vi "Log Binning.vi"(4 "Max Freq":dbl[unit]=1000000000.0 format="%#_6p", 5 "Number Elements":u32=200, 6 "Frequencies":dbl[](array[numeric]), 7 "Spectrum":dbl[](array[numeric])) -> (2 "Frequencies Binned":dbl[](array[numeric]), 3 "Spectrum Binned":dbl[](array[numeric]))   [LabVIEW 2010]
panel:
  out "Log Range":dbl[](array[numeric])=[nan, nan, nan, nan, nan, nan, nan, nan, nan, nan, nan, nan, nan, nan, nan, nan, nan, nan, nan, nan, nan, nan, nan, nan, nan, nan, nan, nan, nan, nan, nan, nan, nan, nan, nan, nan, nan, nan, nan, nan, nan, nan, nan, nan, nan, nan, nan, nan, nan, nan, nan, nan, nan, nan, nan, nan, nan, nan, nan, nan, nan, nan, nan, nan, nan, nan, nan, nan, nan, nan, nan, nan, nan, nan, nan, nan, nan, nan, nan, nan, nan, nan, nan, nan, nan, nan, nan, nan, nan, nan, nan, nan, nan, nan, nan, nan, nan, nan, nan, nan, nan, nan, nan, nan, nan, nan, nan, nan, nan, nan, nan, nan, nan, nan, nan, nan, nan, nan, nan, nan, nan, nan, nan, nan, nan, nan, nan, nan, nan, nan, nan, nan, nan, nan, nan, nan, nan, nan, nan, nan, nan, nan, nan, nan, nan, nan, nan, nan, nan, nan, nan, nan, nan, nan, nan, nan, nan, nan, nan, nan, nan, nan, nan, nan, nan, nan, nan, nan, nan, nan, nan, nan, nan, nan, nan, nan, nan, nan, nan, nan, nan, nan, nan, nan, nan, nan, nan, nan, nan, nan, nan, nan, nan, nan, nan, nan, nan, nan, nan, nan]
  out "XY Graph":cluster{dbl[], dbl[]}[](graph)
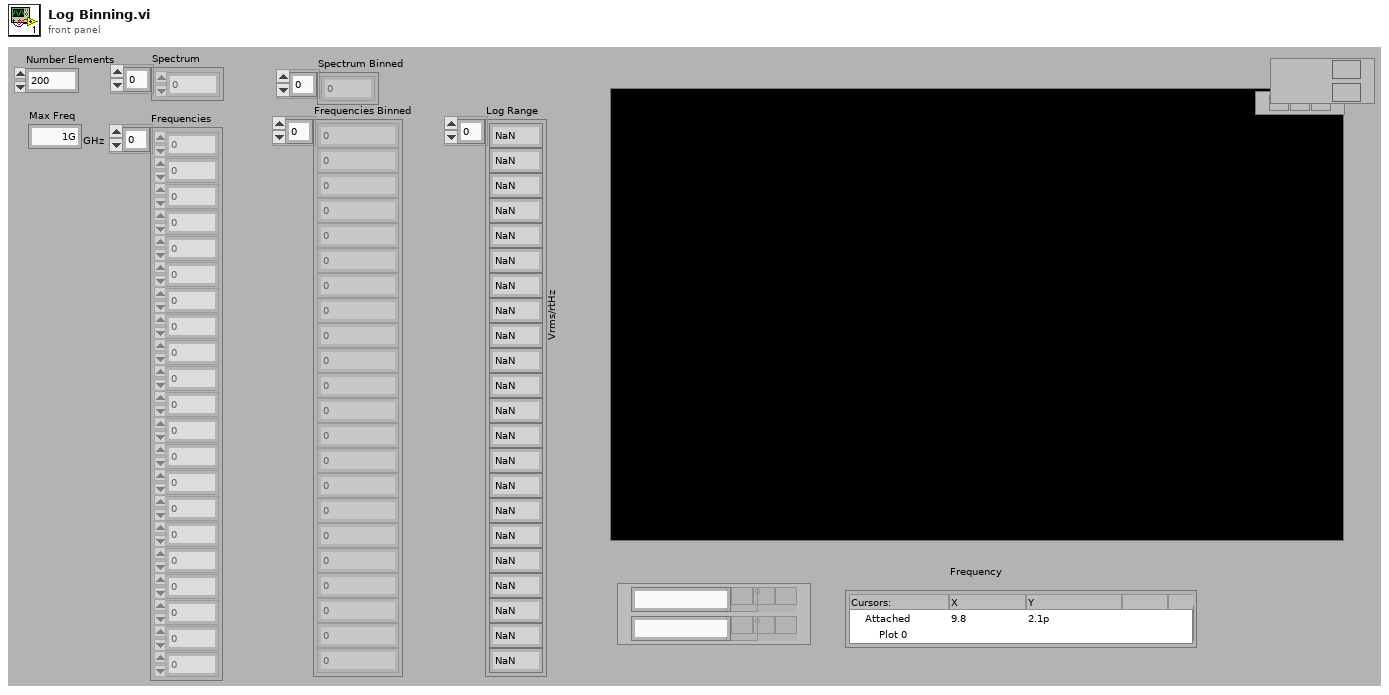
[diagram p1: front panel]
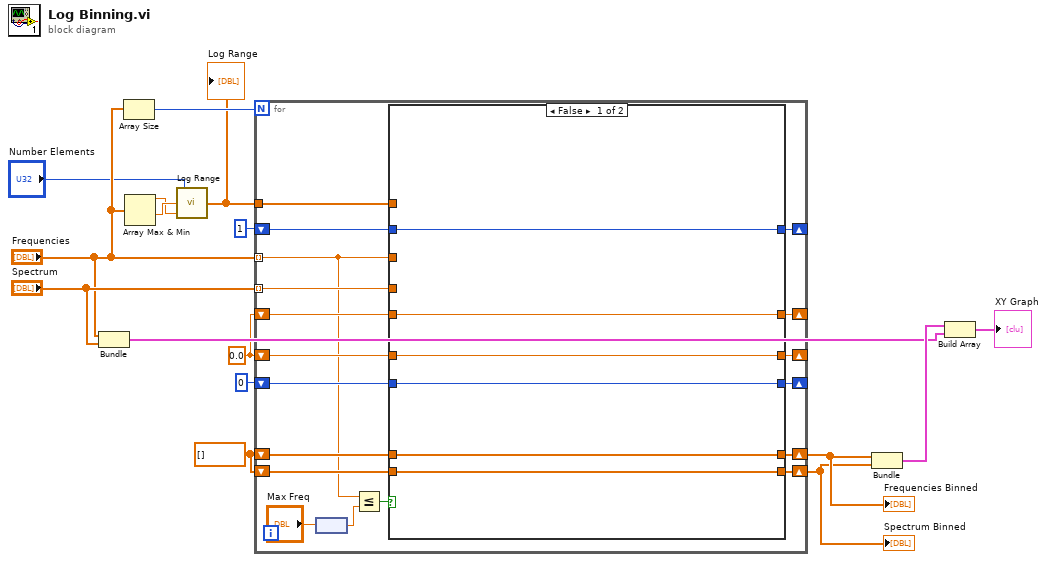
[diagram p0: block diagram]
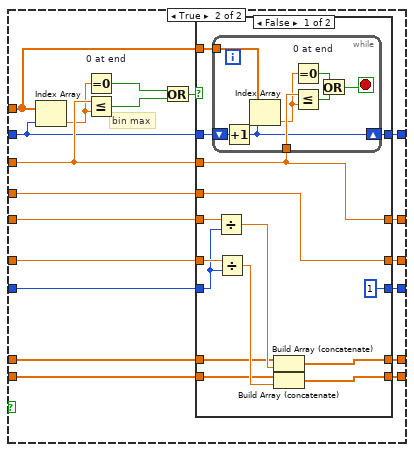
[diagram p2: hidden frame]
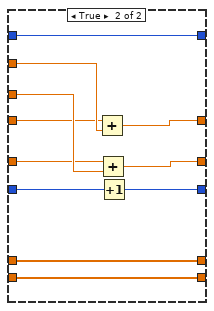
[diagram p3: hidden frame]
diagram:
  w4 = dbl[] []
  w5 = 0.0
  n1 = Bundle("Frequencies"="Frequencies", "Spectrum"="Spectrum") -> (w13:cluster{"Frequencies":dbl[], "Spectrum":dbl[]})  [unwired: 1 out]
  n2 = Array Size(array="Frequencies") -> (size(s)=w12:i32)
  n3 = Array Max & Min(array="Frequencies") -> (max value=w9:dbl, min value=w10:dbl)  [unwired: 2 out]
  n4 = call "Log Range.vi"("Max"=w9, "Min"=w10, "Number Elements"="Number Elements") -> ("Log Range"=w11:dbl[])
  "Log Range" <- w11
  n5 = for {
    N: w12 -> [_]
    tunnel: "Frequencies" -> [w20] mode=indexing
    tunnel: "Spectrum" -> [w34] mode=indexing
    tunnel: w11 -> [w21]
    shift-right: [w22] -> _
    shift-left: u32 1 ("size(s)") -> [w23]
    shift-right: [w28] -> _
    shift-left: u32 0 ("size(s)") -> [w29]
    shift-right: [w32] -> _
    shift-left: w5 -> [w33]
    shift-right: [w31] -> _
    shift-left: w5 -> [w30]
    shift-right: [w27] -> w3
    shift-left: w4 -> [w26]
    shift-right: [w25] -> w2
    shift-left: w4 -> [w24]
    n6 = node("Max Freq") -> (w17:dbl)
    n7 = Less Or Equal?(x=w20, y=w17) -> (x <= y?=w19:bool)
    n8 = case shown="False" w19 {
      tunnel: w20 -> [_ w59]
      tunnel: w34 -> [_ w58]
      tunnel: w33 -> [w39 w57]
      tunnel: [w39 w56] -> w32
      tunnel: [w38 w55] -> w31
      tunnel: w30 -> [w38 w54]
      tunnel: w29 -> [w37 w53]
      tunnel: [w37 w52] -> w28
      tunnel: [w36 w51] -> w27
      tunnel: w26 -> [w36 w50]
      tunnel: [w35 w49] -> w25
      tunnel: w24 -> [w35 w48]
      tunnel: w23 -> [w40 w47]
      tunnel: [w40 w46] -> w22
      tunnel: w21 -> [_ w45]
      frame False {
      }
      frame True {
        # "bin max"
        n9 = Index Array(array=w45, index=w47) -> (element=w41:dbl)
        n10 = Equal To 0? "0 at end"(x=w41) -> (x = 0?=w42:bool)
        n11 = Less Or Equal?(x=w59, y=w41) -> (x <= y?=w44:bool)
        n12 = Or(x=w42, y=w44) -> (x .or. y?=w43:bool)
        n13 = case shown="False" w43 {
          tunnel: w59 -> [w61 w92]
          tunnel: w58 -> [w62 w93]
          tunnel: w57 -> [w73 w91]
          tunnel: [w61 w90] -> w56
          tunnel: [w62 w89] -> w55
          tunnel: w54 -> [w72 w88]
          tunnel: w53 -> [w71 w87]
          tunnel: [u32 1 ("size(s)") w86] -> w52
          tunnel: [w68 w85] -> w51
          tunnel: w50 -> [w67 w85]
          tunnel: [w66 w84] -> w49
          tunnel: w48 -> [w65 w84]
          tunnel: w47 -> [w64 w83]
          tunnel: [w63 w83] -> w46
          tunnel: w45 -> [w60 _]
          frame False {
            n14 = while {
              tunnel: w61 -> [w81]
              tunnel: w60 -> [w80]
              shift-right: [w79] -> w63
              shift-left: w64 -> [w82]
              stop <- w76 stop-if-true
              n15 = Increment(x=w82) -> (x+1=w79:u32)
              n16 = Index Array(array=w80, index=w79) -> (element=w75:dbl)
              n17 = Equal To 0? "0 at end"(x=w75) -> (x = 0?=w77:bool)
              n18 = Less Or Equal?(x=w81, y=w75) -> (x <= y?=w78:bool)
              n19 = Or(x=w77, y=w78) -> (x .or. y?=w76:bool)
            }
            n20 = Divide ("Average Freq")(x=w73, y=w71) -> (x/y=w69:dbl)
            n21 = Divide ("Average Signal")(x=w72, y=w71) -> (x/y=w70:dbl)
            n22 = Build Array (concatenate)(w67, w69) -> (w68:dbl[])
            n23 = Build Array (concatenate)(w65, w70) -> (w66:dbl[])
          }
          frame True {
            n24 = Add(x=w91, y=w92) -> (x+y=w90:dbl)
            n25 = Add(x=w88, y=w93) -> (x+y=w89:dbl)
            n26 = Increment(x=w87) -> (x+1=w86:u32)
          }
        }
      }
    }
  }
  "Spectrum Binned" <- w2
  "Frequencies Binned" <- w3
  n27 = Bundle(w3, w2) -> (w16:cluster{dbl[], dbl[]})  [unwired: 1 out]
  n28 = Build Array(w16, w13) -> (→"XY Graph":cluster{"Frequencies":dbl[], "Spectrum":dbl[]}[])
